vi "TCP Connection Lost.vi"(8 "error in (no error)":errorcluster, 10 "Connection GUID":string, 11 "tWorkerController in":refnum<class "tWorkerController.lvclass">) -> (0 "error out":errorcluster, 3 "tWorkerController out":refnum<class "tWorkerController.lvclass">)   [LabVIEW 2013, in "tWorkerController.lvlib" / "tWorkerController.lvclass"]
uses:
  tWorkerController.lvclass
  <vilib>/ActorFramework/Actor/Actor.lvclass/Actor.ctl
  LVAutomationListener/msgs/Log Event Msg/Log Event Msg.lvclass/Log Event Msg.ctl
  <vilib>/ActorFramework/Message Enqueuer/Message Enqueuer.lvclass/Message Enqueuer.ctl
  <vilib>/ActorFramework/Message Enqueuer/Enqueue.vi
  <vilib>/ActorFramework/Message Priority Queue/Priority Enqueue.vi
  LVAutomationListener/msgs/Log Event Msg/Log Event Msg.lvclass
  <vilib>/ActorFramework/Actor/Actor.lvclass
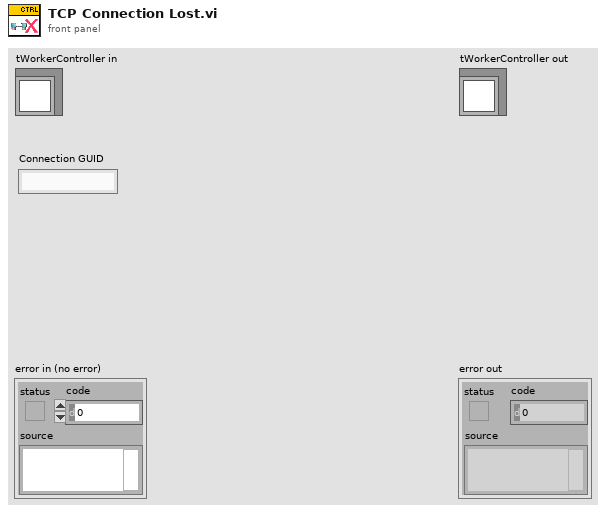
[diagram p1: front panel]
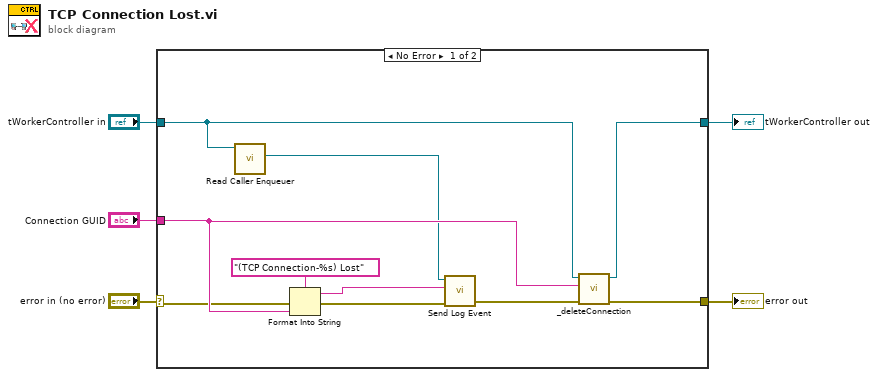
[diagram p0: block diagram]
diagram:
  n1 = case shown="No Error" "error in (no error)" {
    selector: "error in (no error)" -> [w6 w17]
    tunnel: [w14 w17] -> w4
    tunnel: [w15 w16] -> w2
    tunnel: "tWorkerController in" -> [w10 w16]
    tunnel: "Connection GUID" -> [w11 _]
    frame No Error {
      n2 = call <vilib>:"Read Caller Enqueuer.vi"("Actor"=w10) -> ("Caller Enqueuer"=w9:refnum<class "Message Enqueuer.lvclass">)  [unwired: 10 in]
      n3 = Format Into String(format string="(TCP Connection-%s) Lost", error in=w6, w11) -> (resulting string=w7:string, error out=w13:errorcluster)  [unwired: 1 in]
      n4 = call "Send Log Event.vi"("error in (no error)"=w13, "Event Text"=w7, "Message Enqueuer"=w9) -> ("error out"=w8:errorcluster)  [unwired: 7 in, 1 out]
      n5 = call "_deleteConnection.vi"("error in (no error)"=w8, "GUID"=w11, "tWorkerController in"=w10) -> ("error out"=w14:errorcluster, "tWorkerController out"=w15:refnum<class "tWorkerController.lvclass">)  [unwired: 5 in, 2 out]
    }
    frame Error {
    }
  }
  "error out" <- w4
  "tWorkerController out" <- w2
